vi "Get Path Distance.vi"(1 "Filepath":path, 2 "Folder Path":path) -> (0 "Distance":i32)   [LabVIEW 2022 SP3]
doc: "This VI takes a Folder Path and a Filepath as inputs and returns a Distance as output.\n\n - A distance of 0 means that the Filepath points to a file in the same folder as the Folder Path.\n - A distance of 1 means that the Filepath is in a subfolder of the Folder.\n - A distance of 2 means that the file is in a subfolder of a subfolder (two levels down)\n - A distance of 3 means that the file is in a subfolder of a subfolder of a subfolder (three levels down). And so on.\n - A distance of -1 means that the File is not inside the folder hierarchy.\n\nExample 1\nFolder Path = \"C:\\Power Supply Library\"\nFilepath = \"C:\\Power Supply Library\\Turn PSU On.vi\"\nDistance = 0\n\nExample 2\nFolder Path = \"C:\\Power Supply Library\"\nFilepath = \"C:\\Power Supply Library\\Basic Functions\\Turn PSU On.vi\"\nDistance = 1\n\nExample 3\nFolder Path = \"C:\\Power Supply Library\\Basic Functions\"\nFilepath = \"D:\\Utilities\\Turn PSU On.vi\"\nDistance = -1"
panel:
  out "Iteration":i32
  # "Development\nControls or indicators that are useful for development or testing, but which are not outputs of the VI."
  # "Input\nInputs to the VI"
  # "Output\nOutputs of the VI"
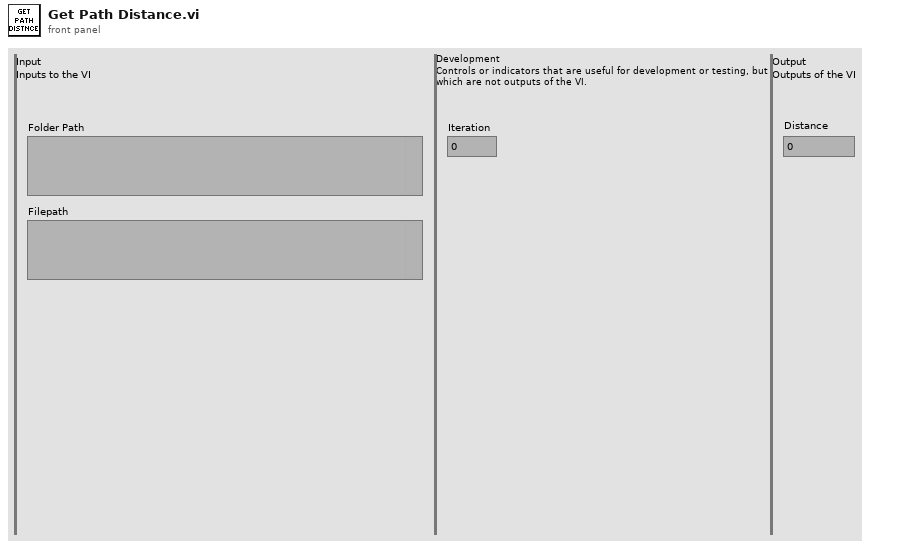
[diagram p1: front panel]
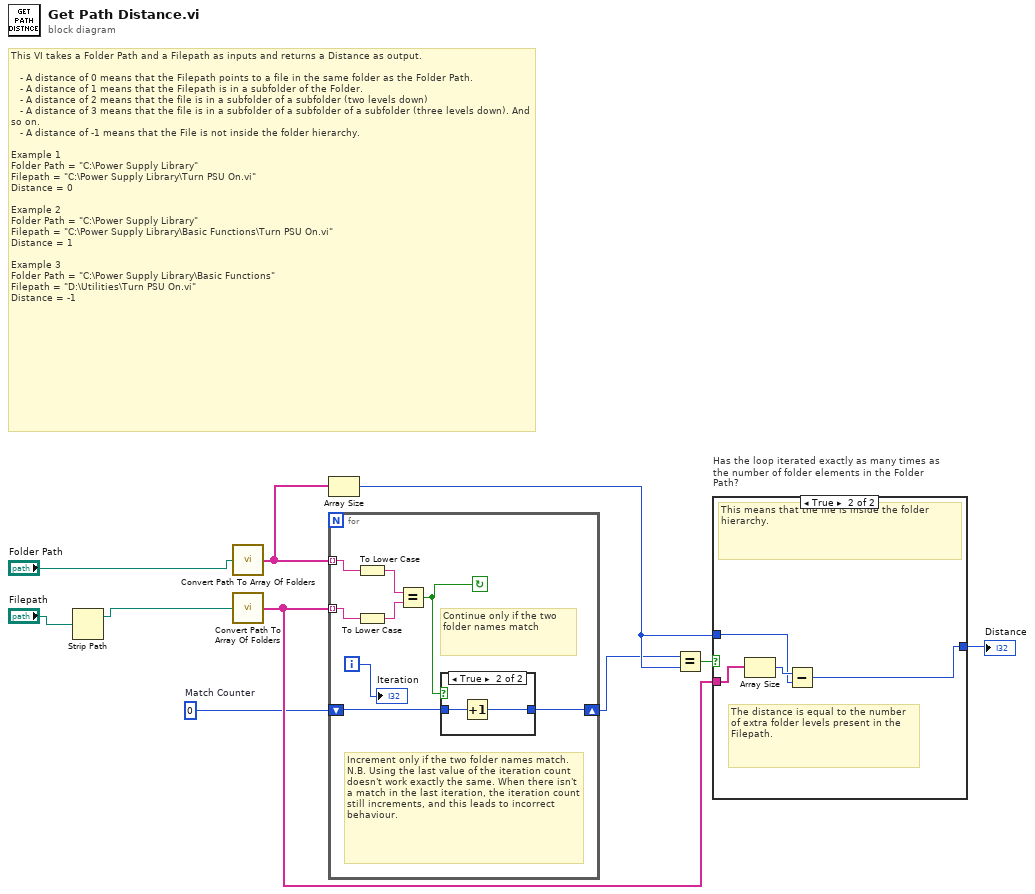
[diagram p0: block diagram]
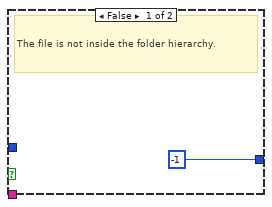
[diagram p2: hidden frame]
diagram:
  w2 = 0  # Match Counter
  # "This VI takes a Folder Path and a Filepath as inputs and returns a Distance as output.\n\n   - A distance of 0 means that the Filepath points to a file in the same folder as the Folder Path.\n   - A distance of 1 means that the Filepath is in a subfolder of the Folder.\n   - A distance of 2 means that the file is in a subfolder of a subfolder (two levels down)\n   - A distance of 3 means that the file is in a subfolder of a subfolder of a subfolder (three levels down). And so on.\n   - A distance of -1 means that the File is not inside the folder hierarchy.\n\nExample 1\nFolder Path = \"C:\\Power Supply Library\"\nFilepath = \"C:\\Power Supply Library\\Turn PSU On.vi\"\nDistance = 0\n\nExample 2\nFolder Path = \"C:\\Power Supply Library\"\nFilepath = \"C:\\Power Supply Library\\Basic Functions\\Turn PSU On.vi\"\nDistance = 1\n\nExample 3\nFolder Path = \"C:\\Power Supply Library\\Basic Functions\"\nFilepath = \"D:\\Utilities\\Turn PSU On.vi\"\nDistance = -1"
  n1 = Strip Path(path="Filepath") -> (stripped path=w8:path)  [unwired: 1 out]
  n2 = call "Convert Path To Array Of Folders.vi"("Folder Path"="Folder Path") -> ("Individual Folders"=w7:string[])
  n3 = call "Convert Path To Array Of Folders.vi"("Folder Path"=w8) -> ("Individual Folders"=w4:string[])
  n4 = Array Size(array=w7) -> (size(s)=w3:i32)
  n5 = for {
    tunnel: w7 -> [w17] mode=indexing
    tunnel: w4 -> [w16] mode=indexing
    shift-right: [w12] -> w1
    shift-left: w2 -> [w13]
    i -> [w18]
    stop <- w11 continue-if-true
    # "Increment only if the two folder names match. N.B. Using the last value of the iteration count doesn't work exactly the same. When there isn't a match in the last iteration, the iteration count still increments, and this leads to incorrect behaviour."
    # "Continue only if the two folder names match"
    n6 = To Lower Case(string=w17) -> (all lower case string=w15:string)
    n7 = To Lower Case(string=w16) -> (all lower case string=w14:string)
    n8 = Equal?(x=w15, y=w14) -> (x = y?=w11:bool)
    n9 = case shown="True" w11 {
      tunnel: w13 -> [w19 w21]
      tunnel: [w19 w20] -> w12
      frame False {
      }
      frame True {
        n10 = Increment(x=w21) -> (x+1=w20:i32)
      }
    }
    "Iteration" <- w18
  }
  n11 = Equal?(x=w1, y=w3) -> (x = y?=w6:bool)
  n12 = case "Has the loop iterated exactly as many times as the number of folder elements in the Folder Path?" shown="True" w6 {
    tunnel: [-1 w23] -> w5
    tunnel: w4 -> [_ w26]
    tunnel: w3 -> [_ w24]
    frame False {
      # "The file is not inside the folder hierarchy."
    }
    frame True {
      # "The distance is equal to the number of extra folder levels present in the Filepath."
      # "This means that the file is inside the folder hierarchy."
      n13 = Array Size(array=w26) -> (size(s)=w25:i32)
      n14 = Subtract(x=w25, y=w24) -> (x-y=w23:i32)
    }
  }
  "Distance" <- w5
